vi "DSF.Execution.Runtime.Plugin Manager.Load Plugin Classes.Runtime.vi"(8 "error in (no error)":errorcluster, 10 "Plugin objects":refnum<class>[](array[class]), 11 "Plugin Manager in":refnum<class "DSF.Engine.Runtime.Plugin Manager.lvclass">) -> (0 "error out":errorcluster, 2 "Plugin Runtime Classes":T1, 3 "Plugin Manager out":refnum<class "DSF.Engine.Runtime.Plugin Manager.lvclass">)   [LabVIEW 2016, in "DSF.Engine.lvlib" / "DSF.Engine.Runtime.Plugin Manager.lvclass"]
uses:
  DSF.Engine.Runtime.Plugin Manager.lvclass
  Shared/Typedefs/DSF.Shared.Typedefs.Plugin Classes.Runtime.ctl
  Plugin/DSF.Engine.Runtime.Plugin.lvclass
  DSF.Shared.lvlib
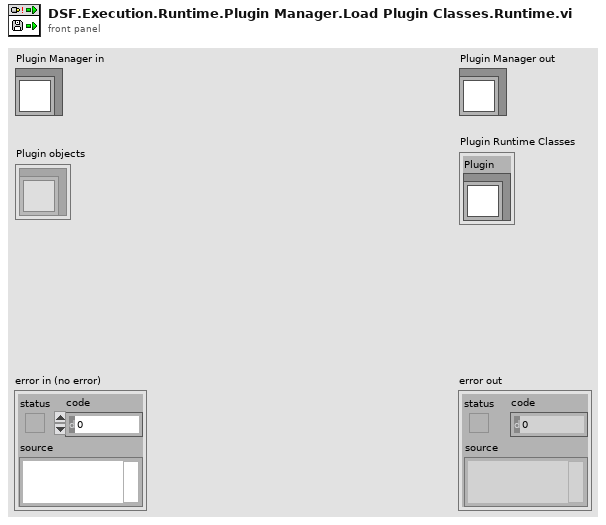
[diagram p1: front panel]
types:
  T1 = typedef "DSF.Shared.lvlib/DSF.Shared.Typedefs.Plugin Classes.Runtime.ctl" = cluster{"Plugin":refnum<class "DSF.Engine.Runtime.Plugin.lvclass">}
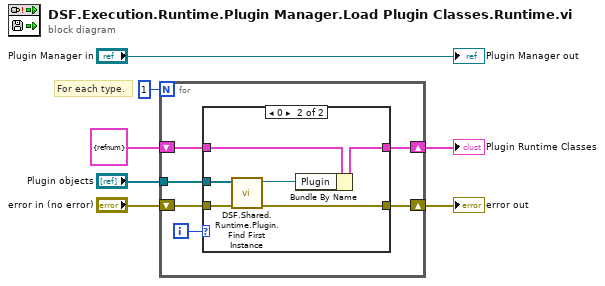
[diagram p0: block diagram]
diagram:
  # "For each type."
  n1 = for {
    N: 1 -> [_]
    shift-right: [w11] -> w2
    shift-left: T1 {"Plugin"=refnum} ("Plugin Runtime Classes") -> [w12]
    shift-right: [w10] -> w3
    shift-left: "error in (no error)" -> [w9]
    tunnel: "Plugin objects" -> [w8]
    i -> [w13]
    n2 = case shown="0" w13 {
      tunnel: w12 -> [w15 w21]
      tunnel: [w15 w20] -> w11
      tunnel: [w14 w17] -> w10
      tunnel: w9 -> [w14 w19]
      tunnel: w8 -> [_ w18]
      frame -1, Default {
      }
      frame 0 {
        n3 = call "DSF.Shared.Runtime.Plugin.Find First Instance.vi"("error in (no error)"=w19, "objects"=w18) -> ("error out"=w17:errorcluster, "Plugin Runtime"=w16:refnum<class "DSF.Engine.Runtime.Plugin.lvclass">)  [unwired: 7 in, 1 out]
        n4 = Bundle By Name(cluster=w21, "Plugin"=w16) -> (w20:T1)
      }
    }
  }
  "error out" <- w3
  "Plugin Runtime Classes" <- w2
  "Plugin Manager out" <- "Plugin Manager in"
